vi "deney_8.1.vi"() -> ()   [LabVIEW 2018]
panel:
  out "tahmin eski":dbl
  out "SAYI":u16
  in  "Tahmin":u16
  out "BITTI":bool
  out "KALAN":i32=10
  out "MESAJ":string="Tahmin : 0 .. 1023"
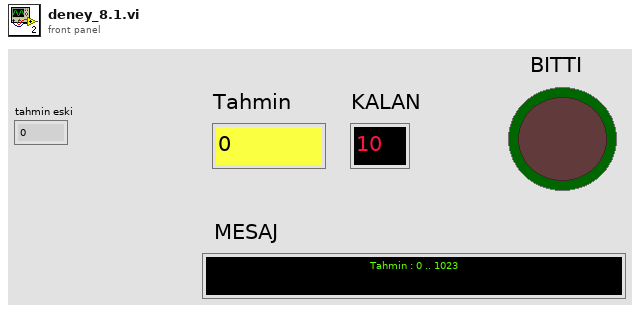
[diagram p1: front panel]
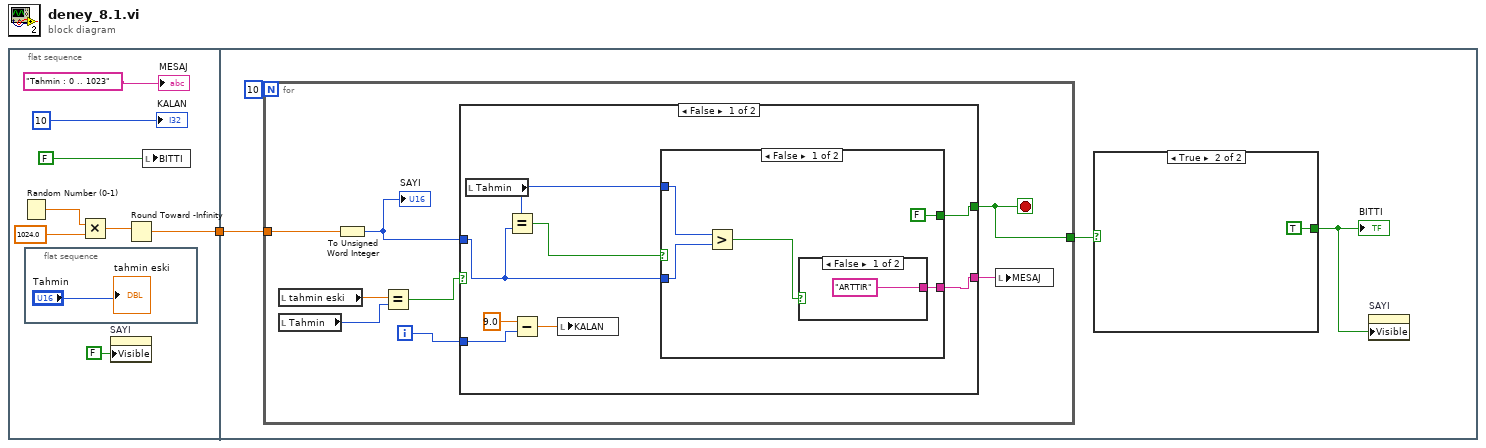
[diagram p0: block diagram]
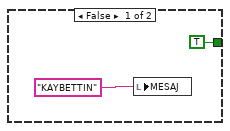
[diagram p2: hidden frame]
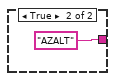
[diagram p3: hidden frame]
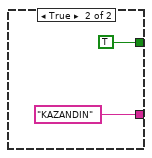
[diagram p4: hidden frame]
diagram:
  n1 = flat-sequence {
    tunnel: [w4] -> w1
    tunnel: w1 -> [w13]
    frame #0 {
      n2 = Random Number (0-1)() -> (number: 0 to 1=w6:dbl)
      n3 = flat-sequence {
        frame #0 {
          "tahmin eski" <- "Tahmin"
        }
      }
      n4 = Multiply(x=w6, y=1024.0) -> (x*y=w5:dbl)
      n5 = property on="SAYI" class="DigNum (strict)"("Visible"=FALSE) -> ()  [unwired: 2 in, 2 out]
      n6 = Round Toward -Infinity(1:w5) -> (0:w4:dbl)
      n7 = local write "BITTI"(FALSE ("BITTI")) -> ()
      "MESAJ" <- "Tahmin : 0 .. 1023"
      "KALAN" <- 10
    }
    frame #1 {
      n8 = for {
        N: 10 -> [_]
        tunnel: w13 -> [w25]
        tunnel: [w21] -> w12
        i -> [w23]
        stop <- w21 stop-if-true
        n9 = local read "tahmin eski"() -> (w20:dbl)
        n10 = local read "Tahmin"() -> (w19:u16)
        n11 = To Unsigned Word Integer(number=w25) -> (unsigned 16bit integer=w24:u16)
        "SAYI" <- w24
        n12 = Equal?(x=w20, y=w19) -> (x = y?=w18:bool)
        n13 = case shown="False" w18 {
          tunnel: w24 -> [w33 _]
          tunnel: w23 -> [w32 _]
          tunnel: [w31 _] -> w22
          tunnel: [w30 _] -> w21
          frame False {
            n14 = local read "Tahmin"() -> (w26:u16)
            n15 = Equal?(x=w26, y=w33) -> (x = y?=w29:bool)
            n16 = Subtract(x=9.0, y=w32) -> (x-y=w27:dbl)
            n17 = local write "KALAN"(w27) -> ()
            n18 = case shown="False" w29 {
              tunnel: w33 -> [w37 _]
              tunnel: w26 -> [w38 _]
              tunnel: [FALSE TRUE] -> w30
              tunnel: [w35 "KAZANDIN" ("MESAJ")] -> w31
              frame False {
                n19 = Greater?(x=w38, y=w37) -> (0:w36:bool)
                n20 = case shown="False" w36 {
                  tunnel: ["ARTTIR" ("MESAJ") "AZALT" ("MESAJ")] -> w35
                  frame False {
                  }
                  frame True {
                  }
                }
              }
              frame True {
              }
            }
          }
          frame True {
          }
        }
        n21 = local write "MESAJ"(w22) -> ()
      }
      n22 = case shown="True" w12 {
        tunnel: [TRUE TRUE] -> w11
        frame False {
          n23 = local write "MESAJ"("KAYBETTIN" ("MESAJ")) -> ()
        }
        frame True {
        }
      }
      "BITTI" <- w11
      n24 = property on="SAYI" class="DigNum (strict)"("Visible"=w11) -> ()  [unwired: 2 in, 2 out]
    }
  }
